vi "Get Motor Pos.vi"(8 "error in (no error)":errorcluster, 11 "VacuumLine in":refnum<class "VacuumLine.lvclass">) -> (0 "error out":errorcluster, 2 "Motor Pos":dbl, 3 "VacuumLine out":refnum<class "VacuumLine.lvclass">)   [LabVIEW 2016, in "Hardware.lvlib" / "VacuumLine.lvlib" / "VacuumLine.lvclass"]
uses:
  <userlib>/Common Components/Hardware/Abstract System/VacuumLine/VacuumLine/VacuumLine.lvclass
  <userlib>/Common Components/Hardware/Abstract System/VacuumLine/VacuumLine/VacuumLine.lvclass/VacuumLine.ctl
  <userlib>/Common Components/Hardware/Motor/Motor/Motor.lvclass
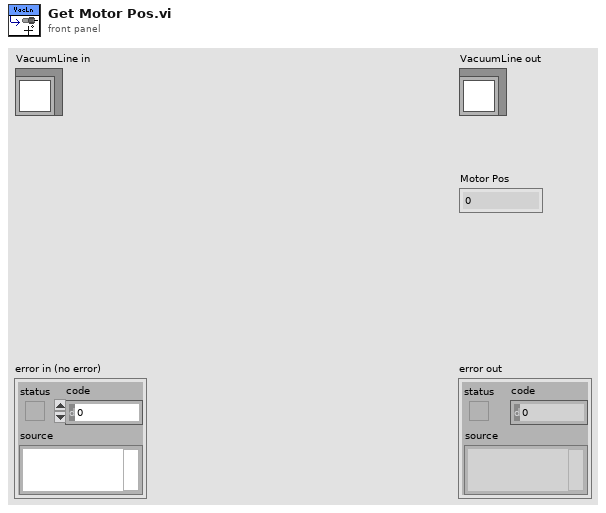
[diagram p1: front panel]
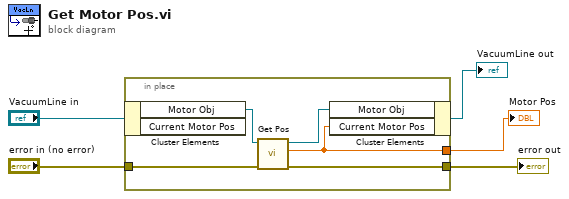
[diagram p0: block diagram]
diagram:
  n1 = in-place {
    in-place-border: "error in (no error)" -> [w10]
    in-place-border: [w9] -> w4
    in-place-border: [w6] -> w3
    n2 = in-place-cluster #1("VacuumLine in") -> ("Motor Obj"=w8:refnum<class "Motor.lvclass">)  [unwired: 1 out]
    n3 = call <userlib>:"Get Pos.vi"("error in (no error)"=w10, "Motor in"=w8) -> ("error out"=w9:errorcluster, "Position in unit mode"=w6:dbl, "Motor out"=w7:refnum<class "Motor.lvclass">)  [unwired: 7 in]
    n4 = in-place-cluster #1("Motor Obj"=w7, "Current Motor Pos"=w6) -> (→"VacuumLine out":refnum<class "VacuumLine.lvclass">)
  }
  "error out" <- w4
  "Motor Pos" <- w3
